vi "SubVI Tester.vi"() -> ()   [LabVIEW 2015]
panel:
  out "Warning Text":string="No Warning"
  out "Warning?":bool
  out "Thermometer":dbl(slide) scale=0.0..100.0
  in  "Min Temperature":dbl=10.0
  in  "Max Temperature":dbl=30.0
  in  "Stop":bool
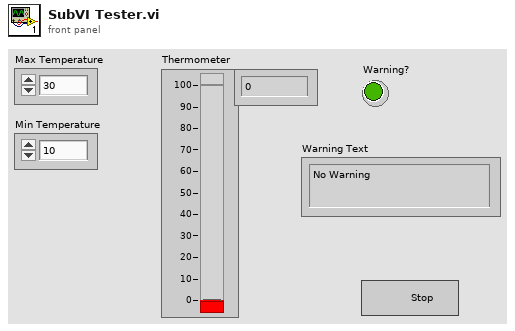
[diagram p1: front panel]
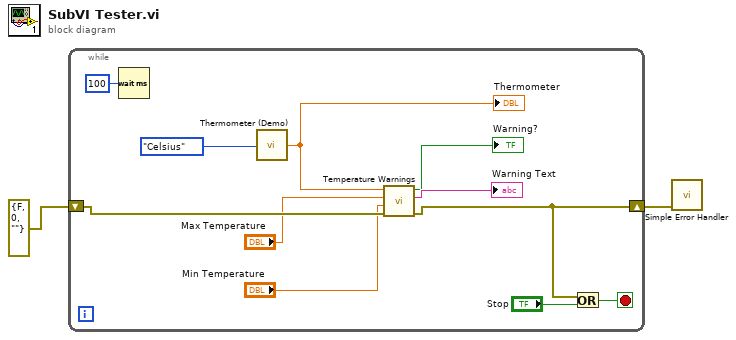
[diagram p0: block diagram]
diagram:
  n1 = while {
    shift-right: [w3] -> w2
    shift-left: errorcluster {"status"=FALSE, "code"=0, "source"=""} ("error in") -> [w9]
    stop <- w11 stop-if-true
    n2 = Wait (ms)(milliseconds to wait=u32 100) -> ()  [unwired: 1 out]
    n3 = call "Thermometer (Demo).vi"("Units (0: Celsius)"=enum16{"Celsius", "Fahrenheit"}."Celsius") -> ("Temperature Value"=w4:dbl)
    "Thermometer" <- w4
    n4 = call "Temperature Warnings.vi"("Error In"=w9, "Min Temperature"="Min Temperature", "Max Temperature"="Max Temperature", "Current Temperature"=w4) -> ("Error Out"=w3:errorcluster, "Warning Text"=→"Warning Text":string, "Warning?"=→"Warning?":bool)  [unwired: 5 in]
    n5 = Or(x=w3, y="Stop") -> (x .or. y?=w11:bool)
  }
  n6 = call <vilib>:"Simple Error Handler.vi"("error in (no error)"=w2) -> ()  [unwired: 4 in, 5 out]
